vi "R_HA Gas Constant of Humid Air (KJ to Kg K).vi"(1 "Gas Presure":dbl[unit]=80000.0 min=80000.0 max=120000.0, 2 "Tceg":dbl[unit], 3 "RH":dbl) -> (0 "R_HA":dbl[unit])   [LabVIEW 2018]
panel:
  out "R_HA\nGas Constant of Humid Air\nR_HA=R*(1+0.608*HR)/M_HA (J/Kg K)":dbl[unit](knob) scale=0.0..1500000.0
  out "Temprature Of Input Air\nKelvin Degree":dbl[unit](slide) scale=273.0..373.0
  out "Tk":dbl[unit]
  out "Temprature Of Input Air\nCentigrade Degree":dbl[unit](slide) scale=0.0..100.0
  out "Humidity of Input Air":dbl(knob) scale=0.0..100.0
  out "R":dbl[unit]
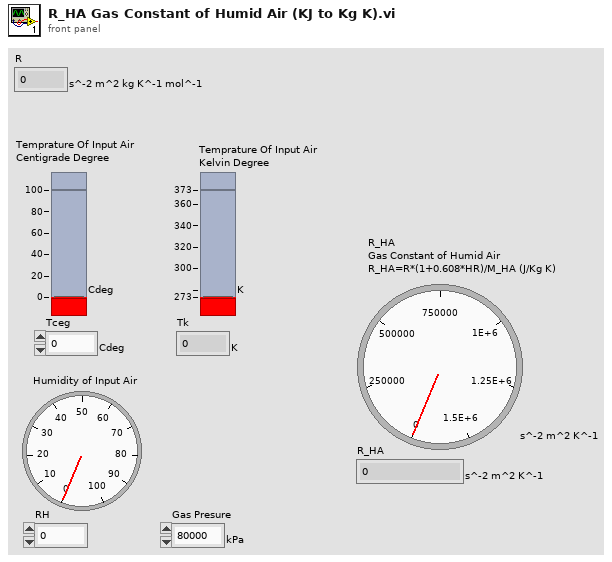
[diagram p1: front panel]
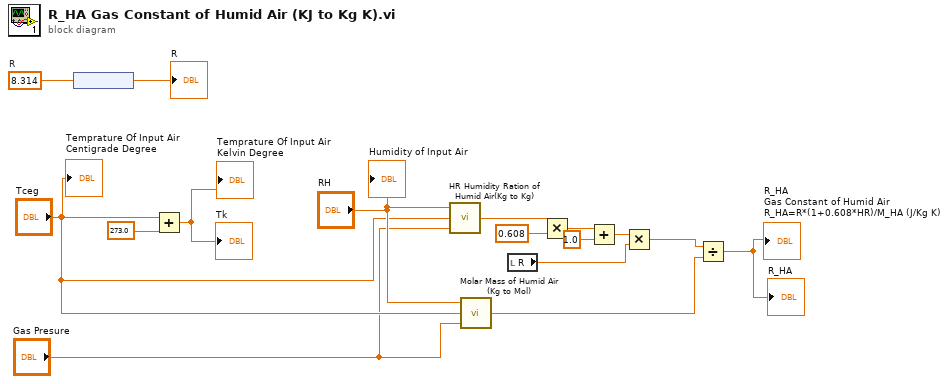
[diagram p0: block diagram]
diagram:
  w16 = 8.314  # R
  n1 = node(w16) -> (→"R":dbl[unit])
  n2 = Add(x="Tceg", y=dbl[unit] 273.0) -> (x+y=→"Tk" →"Temprature Of Input Air\nKelvin Degree":dbl[unit])
  n3 = call "HR Humidity Ration of Humid Air(Kg to Kg).vi"("Gas Presure"="Gas Presure", "Tceg"="Tceg", "RH"="RH") -> ("HR"=w2:dbl)
  n4 = call "Molar Mass of Humid Air (Kg to Mol).vi"("Gas Presure"="Gas Presure", "Tceg"="Tceg", "RH"="RH") -> ("MMH\nMolar Mass of Humid Air (Kg/mol)"=w5:dbl[unit])
  n5 = local read "R"() -> (w6:dbl[unit])
  n6 = Multiply(x=w2, y=0.608) -> (x*y=w10:dbl)
  n7 = Add(x=w10, y=1.0) -> (x+y=w12:dbl)
  n8 = Multiply(x=w12, y=w6) -> (x*y=w8:dbl[unit])
  n9 = Divide(x=w8, y=w5) -> (x/y=→"R_HA\nGas Constant of Humid Air\nR_HA=R*(1+0.608*HR)/M_HA (J/Kg K)" →"R_HA":dbl[unit])
  "Humidity of Input Air" <- "RH"
  "Temprature Of Input Air\nCentigrade Degree" <- "Tceg"
